vi "poumiandatacomb.vi"(6 "数据类型实时小时":string(combo)="-Avg=", 7 "数据值":string[](array[string])=["17.991", "52.06", "45.09", "0.02", "0.03"], 9 "层数":string="1", 10 "数据标识":string="N", 11 "数据类型":string="N") -> (3 "编码输出":string)   [LabVIEW 2016, in "212format_work.lvclass"]
uses:
  212format_work.lvclass
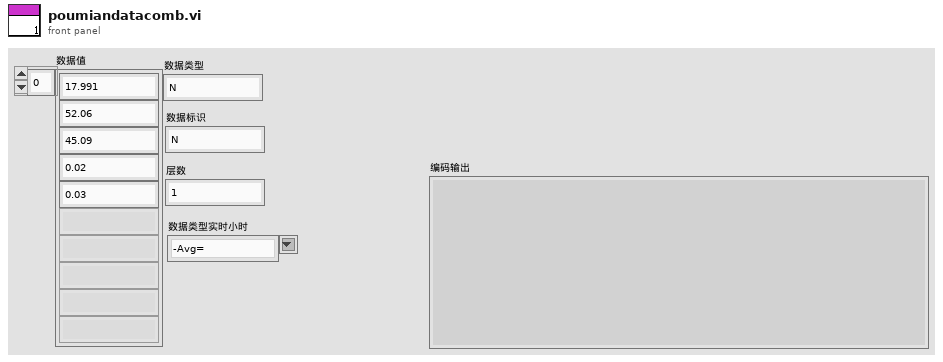
[diagram p1: front panel]
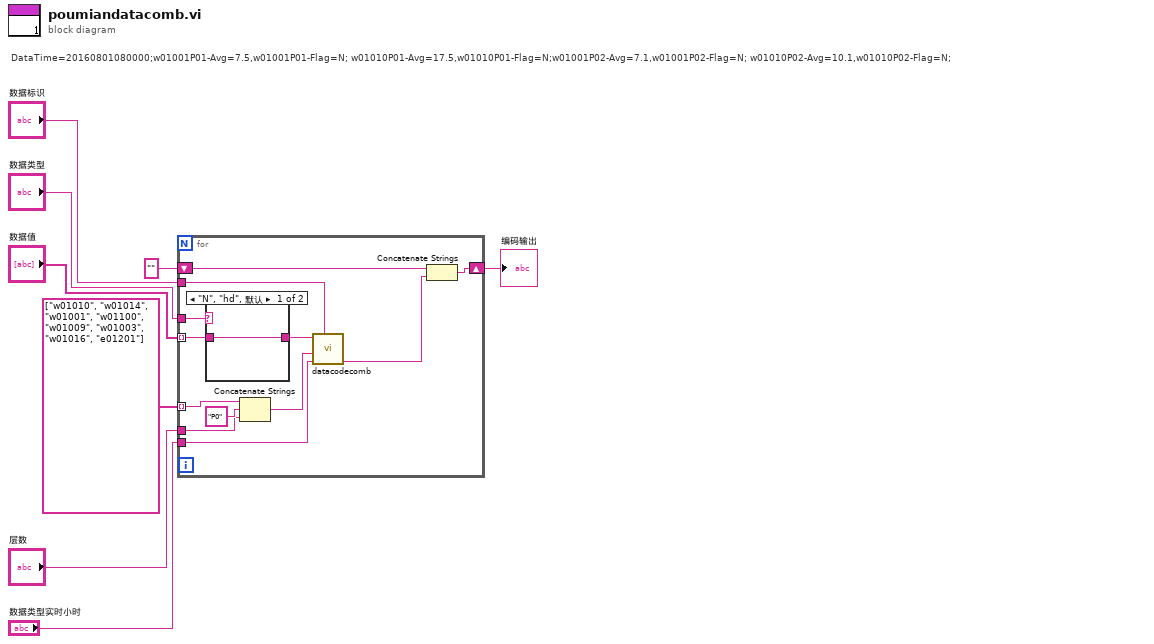
[diagram p0: block diagram]
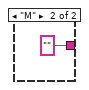
[diagram p2: hidden frame]
diagram:
  # "DataTime=20160801080000;w01001P01-Avg=7.5,w01001P01-Flag=N; w01010P01-Avg=17.5,w01010P01-Flag=N;w01001P02-Avg=7.1,w01001P02-Flag=N; w01010P02-Avg=10.1,w01010P02-Flag=N;"
  n1 = for {
    tunnel: "数据类型" -> [w20]
    tunnel: "层数" -> [w14]
    tunnel: "数据标识" -> [w13]
    tunnel: "数据值" -> [w19] mode=indexing
    shift-right: [w17] -> w5
    shift-left: "" ("编码输出") -> [w18]
    tunnel: string[] ["w01010", "w01014", "w01001", "w01100", "w01009", "w01003", "w01016", "e01201"] -> [w16] mode=indexing
    tunnel: "数据类型实时小时" -> [w11]
    n2 = case shown="\"N\", \"hd\", 默认" w20 {
      tunnel: [w21 ""] -> w12
      tunnel: w19 -> [w21 _]
      frame "N", "hd", Default {
      }
      frame "M" {
      }
    }
    n3 = Concatenate Strings(w16, "P0" ("字符串"), w14) -> (w10:string)
    n4 = call "datacodecomb.vi"("数据标识"=w13, "数据类型"=w11, "污染物编码"=w10, "污染物浓度"=w12) -> ("编码输出"=w9:string)  [unwired: 7 in]
    n5 = Concatenate Strings(w18, w9) -> (w17:string)
  }
  "编码输出" <- w5
